vi "RT_TCP_Listener_Enque.vi"(8 "Error In":errorcluster, 10 "Listener States":T1, 11 "Queue In":refnum<queue>) -> (0 "Error Out":errorcluster, 3 "Queue Out":refnum<queue>)   [LabVIEW 2018]
uses:
  RT_Listener_states.ctl
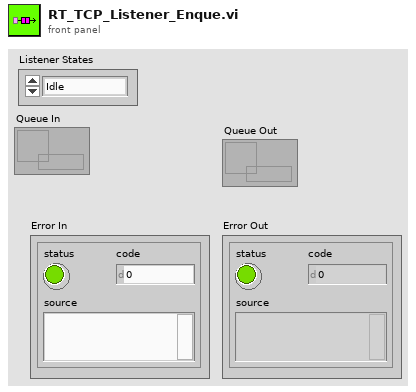
[diagram p1: front panel]
types:
  T1 = typedef "RT_Listener_states.ctl" = enum16{"Idle", "Listen", "Wait", "Exit"}
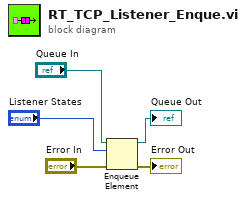
[diagram p0: block diagram]
diagram:
  n1 = Enqueue Element(queue="Queue In", element="Listener States", error in (no error)="Error In") -> (queue out=→"Queue Out":refnum<queue>, error out=→"Error Out":errorcluster)  [unwired: 1 in, 1 out]
